vi "TDMS - File Viewer-Custom.vi"(4 "error in (no error)":errorcluster caption="entrée d'erreur (pas d'erreur)", 7 "file path":path caption="chemin du fichier") -> (0 "error out":errorcluster caption="sortie d'erreur", 3 "file path out":path caption="chemin du fichier en sortie")   [LabVIEW 2015]
doc: "<B>Copyright :</B> (c) 2015 National Instruments. Tous droits réservés.\n\nOuvre le fichier .tdms spécifié dans l'entrée <B>chemin du fichier</B> et présente les données du fichier dans la boîte de dialogue TDMS - Afficheur de fichier."
uses:
  <vilib>/Utility/tdmsutil.llb/fileViewerConfigData.ctl
  <vilib>/Utility/error.llb/DialogType.ctl
  <vilib>/event_ctls.llb/sizeaction.ctl
  <vilib>/event_ctls.llb/panelstate.ctl
  <vilib>/Utility/tdmsutil.llb/TDMSFileViewerLocalizedText.vi
  Instance           1 26Saved   TDMS - File Viewer .vi
panel:
  out "LastXScaleFormat":u8 caption="DernierFormatÉchelleX"
  out "TotalCount":u64 caption="Total"
  out "Temp Configuration":T1 caption="Configuration temp."
  in  "LastTopLeftValue":u64 caption="DernièreValeurSupGauche"
  out "Resize?":bool caption="Redimensionner ?"
  in  "Help":bool caption="Aide"
  in  "Status":string caption="État"
  in  "Quit":bool caption="Quitter"
  in  "Settings...":bool caption="Paramètres..."
  in  "Properties / Values / Graph":T2(tab) caption="Propriétés / Valeurs / Graphe"
  in  "Properties":i32(listbox) caption="Propriétés"
  in  "Go To":bool caption="Atteindre"
  in  "Scrollbar":u64(c297) caption="Barre de défilement"
  in  "Raw data values":i32(listbox) caption="Valeurs des données brutes"
  out "Waveform Graph":waveform(dbl)[](graph) caption="Graphe"
  in  "File contents":string(tree) caption="Contenu du fichier"
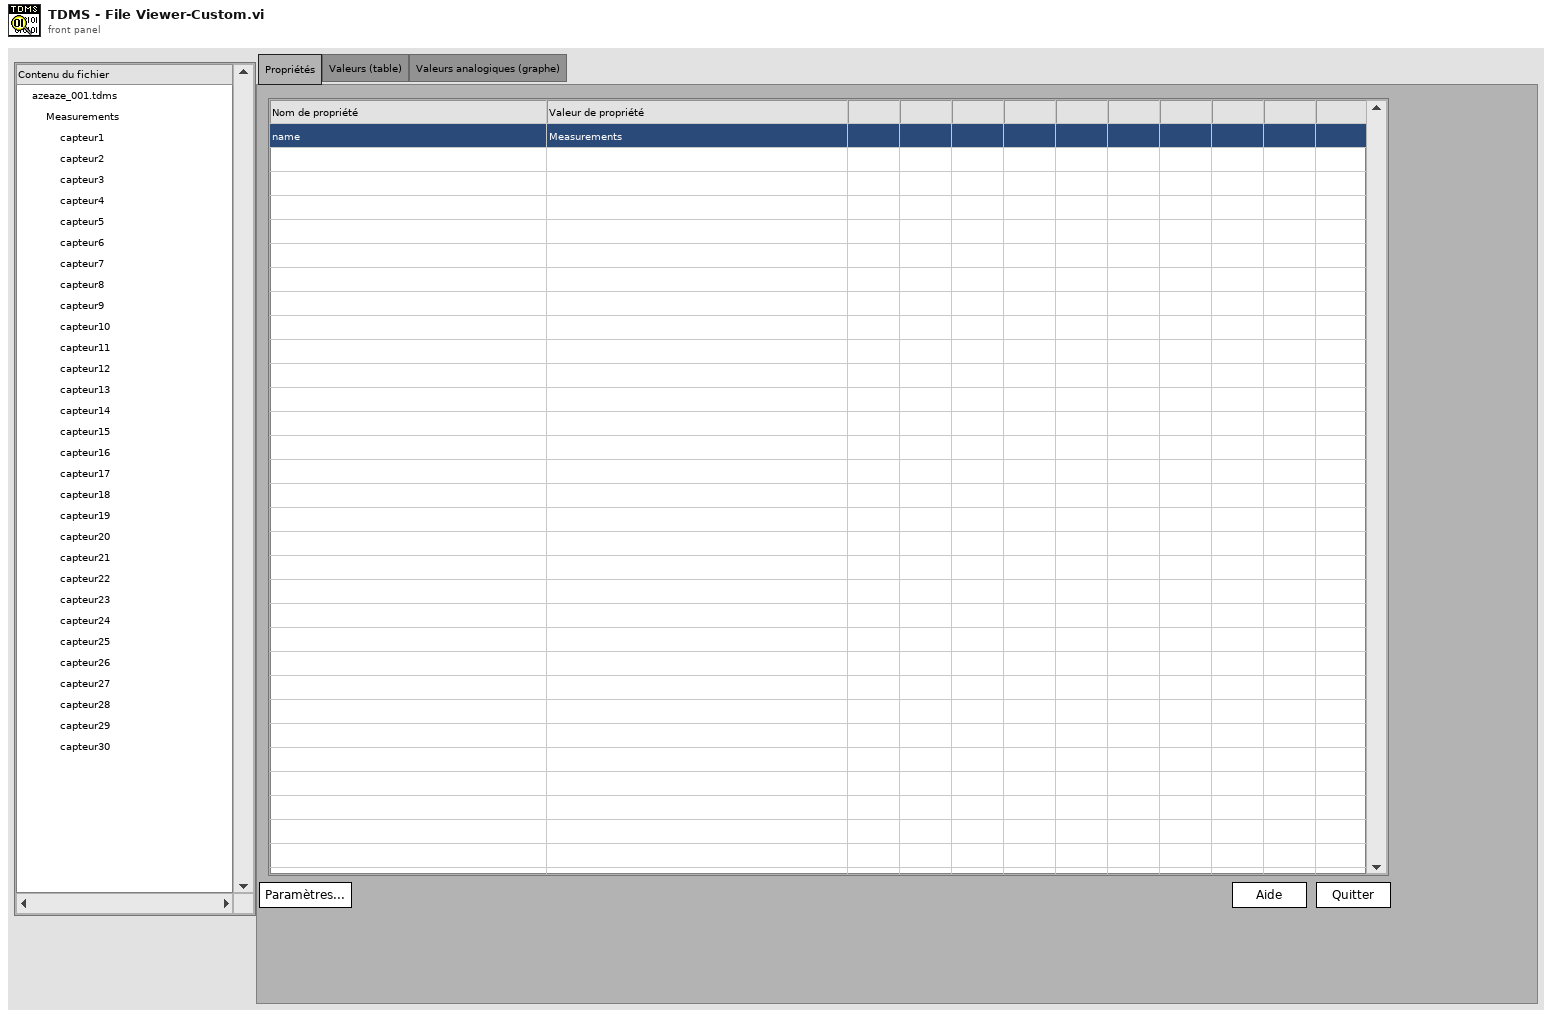
[diagram p1: front panel]
types:
  T1 = typedef "fileViewerConfigData.ctl" = cluster{"Show all (table)":bool, "Show all (graph)":bool, "limit (table)":u64, "limit (graph)":u64, "no show":bool, "start (table)":u64, "start (graph)":u64}
  T2 = enum32{"Properties", "Values (table)", "Analog values (graph)"}
  T3 = enum16{"open", "open or create", "create or replace", "create", "open (read-only)"}
  T4 = cluster{"Tree":refnum<vi>, "Tab Control":refnum<vi>, "property list":refnum<vi>, "raw data list":refnum<vi>, "Waveform Graph":refnum<vi>, "Ok":refnum<vi>, "Ok 2":refnum<vi>, "Ok 3":refnum<vi>, "Ok 4":refnum<vi>, "Scrollbar":refnum<vi>, "Ok 5":refnum<vi>, "TopLeftValue":refnum<vi>, "TotalCount":refnum<vi>}
  T5 = typedef "panelstate.ctl" = enum32{"Standard", "Minimized", "Maximized"}
  T6 = typedef "sizeaction.ctl" = enum32{"Minimized", "Maximized", "Resized"}
  T7 = cluster{"Shift":bool, "Ctrl":bool, "Alt":bool, "Cmd":bool, "Opt":bool}
  T8 = typedef "LVRectTypeDef.ctl" = cluster{"Left":i16, "Top":i16, "Right":i16, "Bottom":i16}
  T9 = typedef "LVRowAndColumnUnsignedTypeDef.ctl" = cluster{"Row":u32, "Column":u32}
  T10 = typedef "DialogType.ctl" = u16
  T11 = typedef "eventvkey.ctl" = enum16{"ASCII", "Enter", "Return", "Shift", "Ctrl", "Alt", "Cmd", "Opt", "Caps", "NumLock", "Clear", "Break", "Up", "Down", "Left", "Right", "Insert", "Delete", "Home", "End", "PageUp", "PageDown", "Escape", "Help", "Pause", "ScrollLock", "F1", "F2", "F3", "F4", "F5", "F6", "F7", "F8", "F9", "F10", "F11", "F12", "F13", "F14", "F15", "F16", "F17", "F18", "F19", "F20", "F21", "F22", "F23", "F24", "Play", "VolumeUp", "VolumeDown", "Mute", "Two Byte Char"}
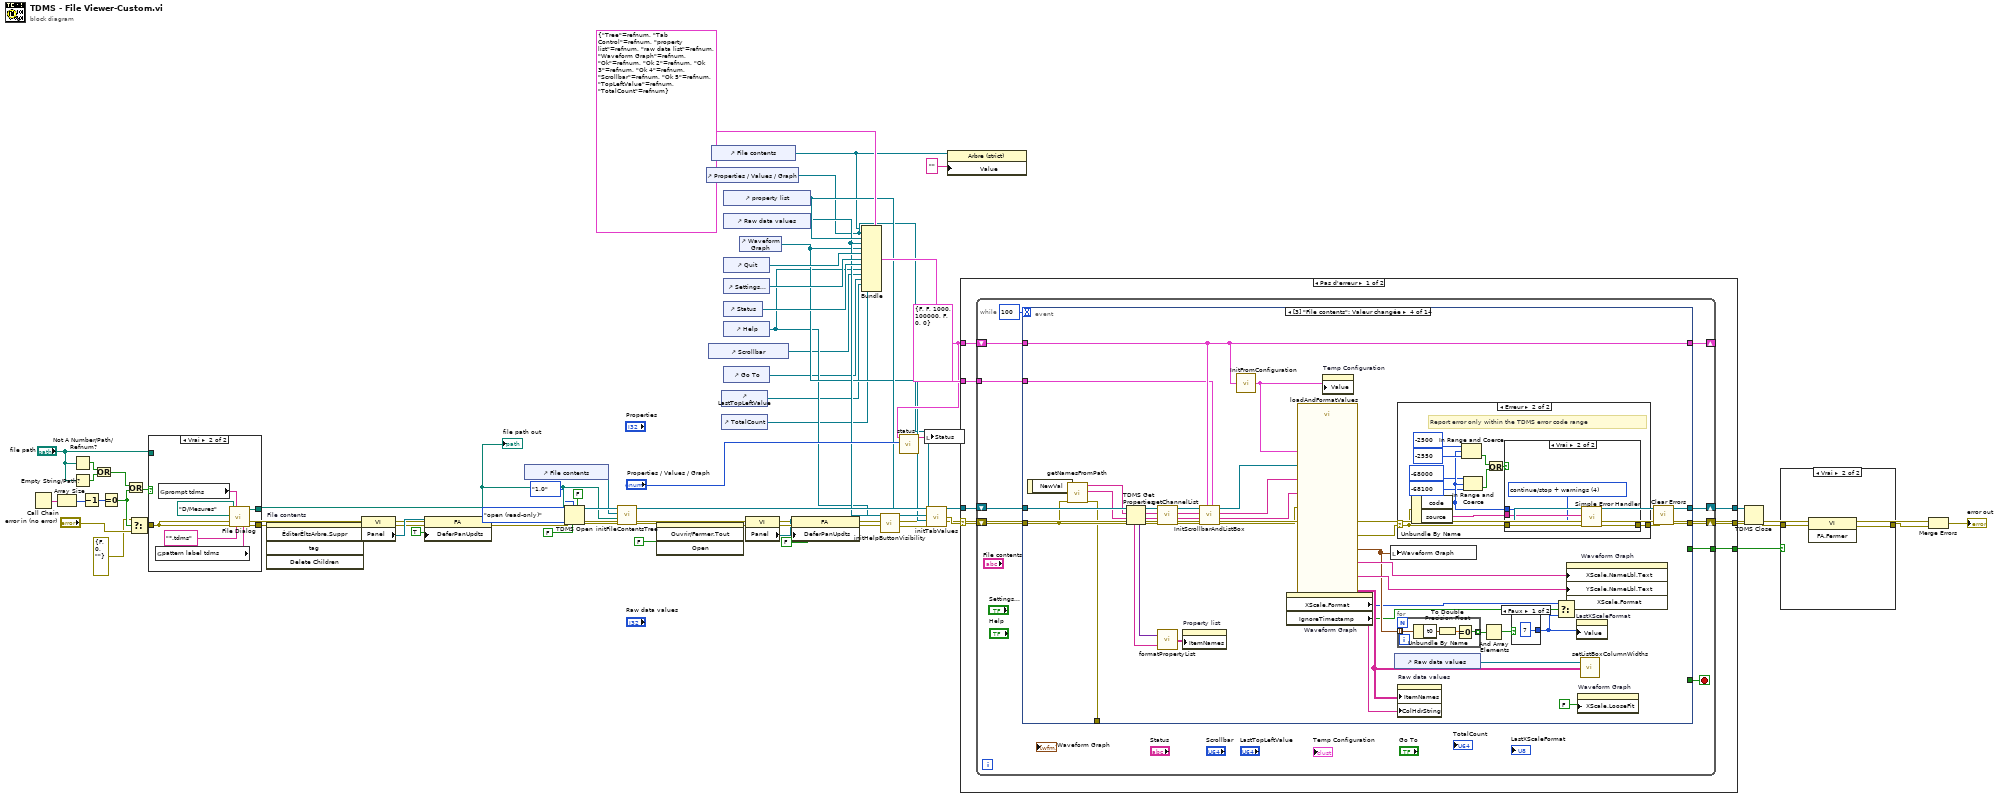
[diagram p0: block diagram]
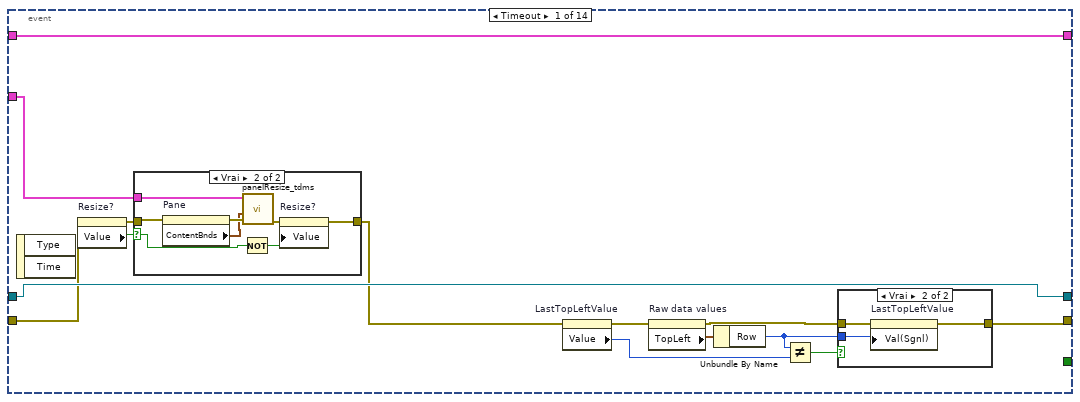
[diagram p3: hidden frame]
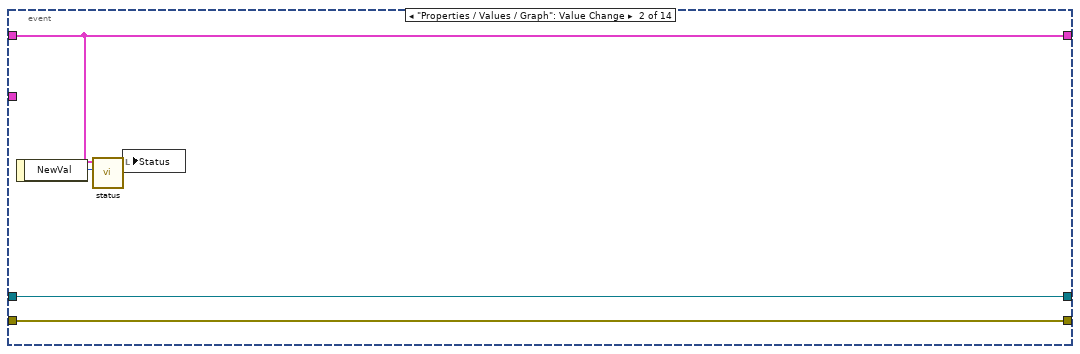
[diagram p6: hidden frame]
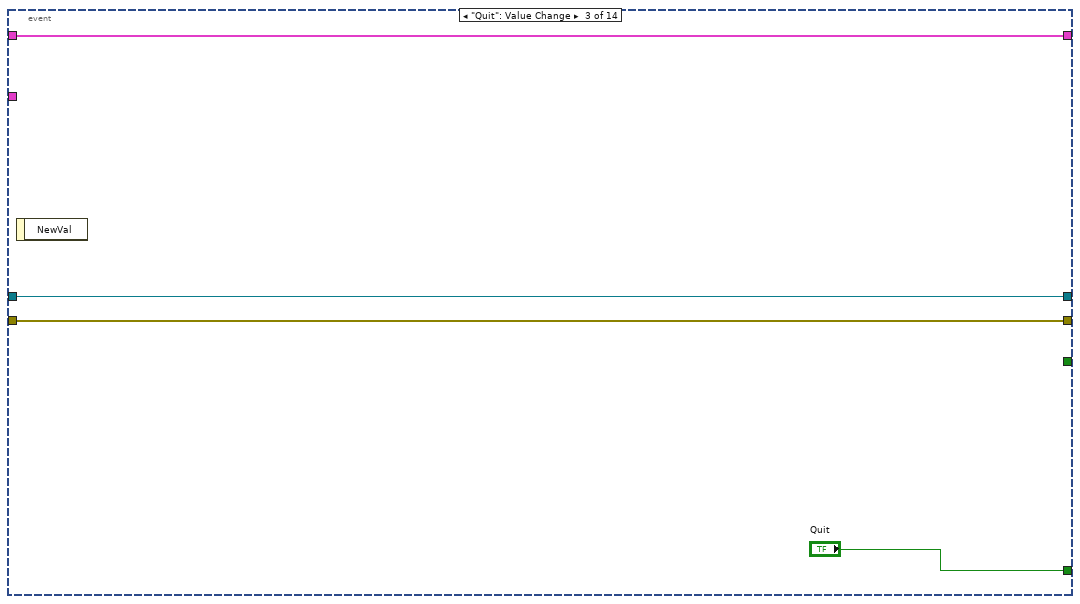
[diagram p7: hidden frame]
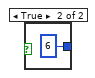
[diagram p8: hidden frame]
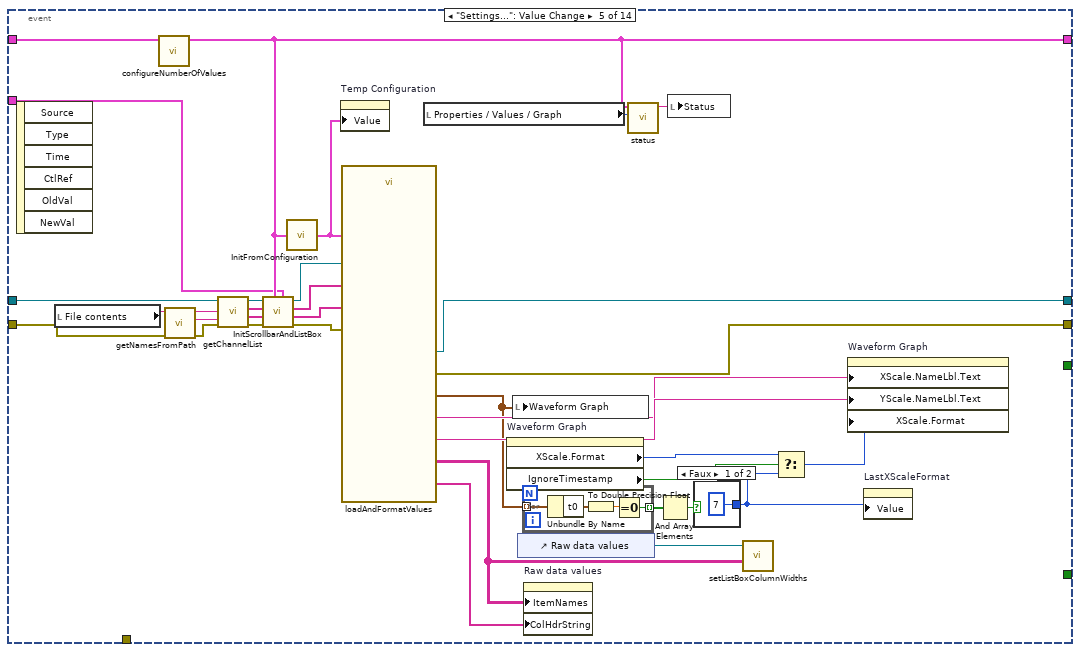
[diagram p11: hidden frame]
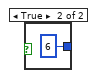
[diagram p12: hidden frame]
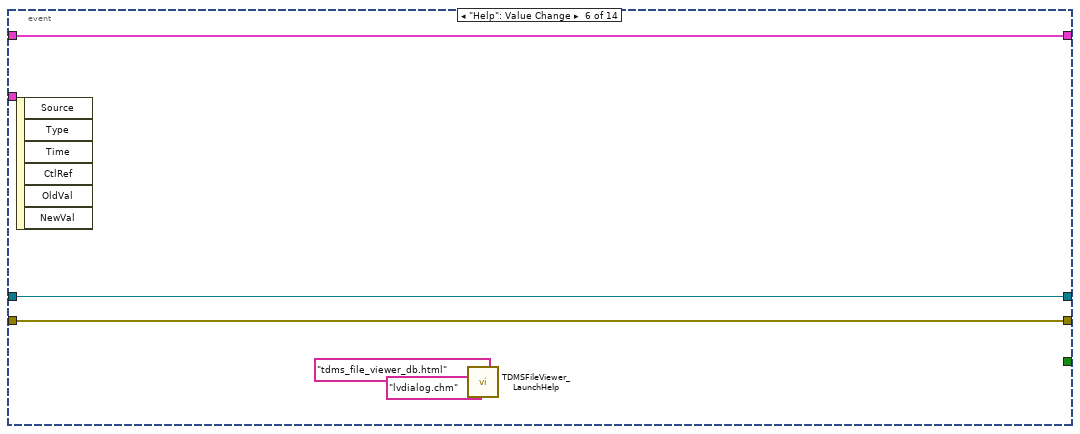
[diagram p13: hidden frame]
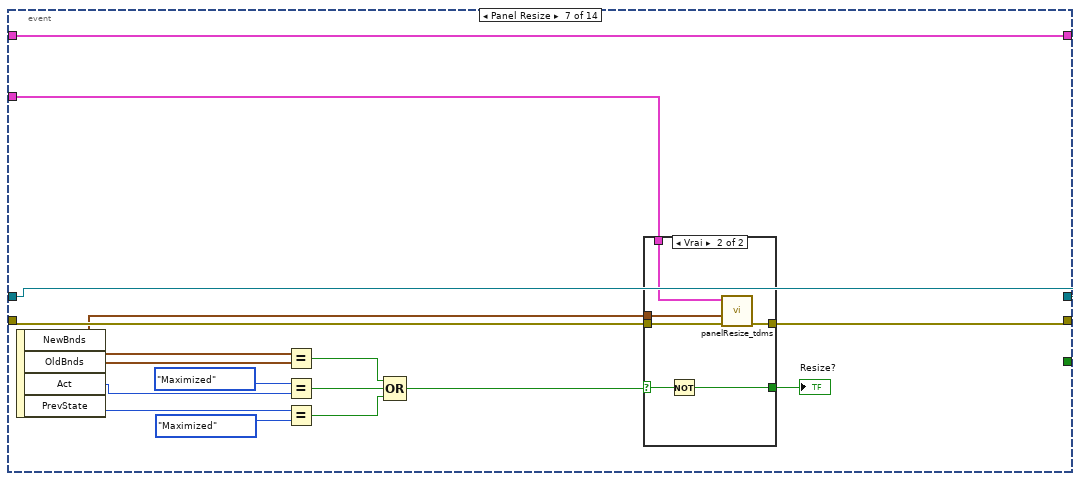
[diagram p14: hidden frame]
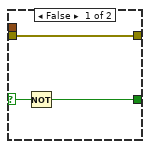
[diagram p15: hidden frame]
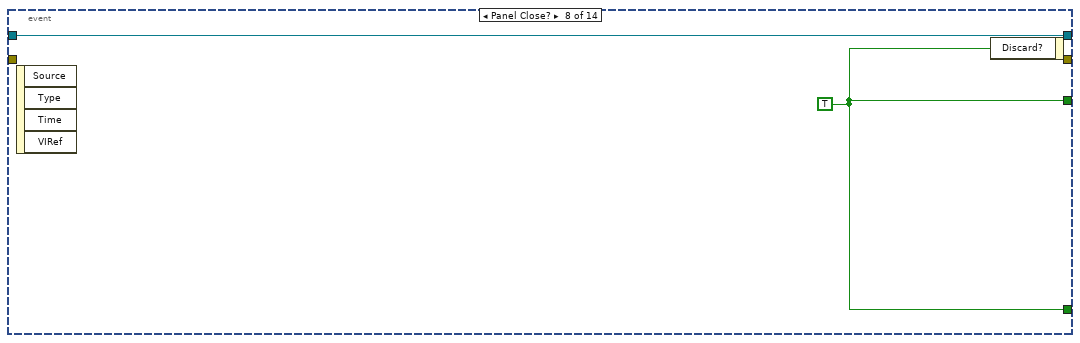
[diagram p16: hidden frame]
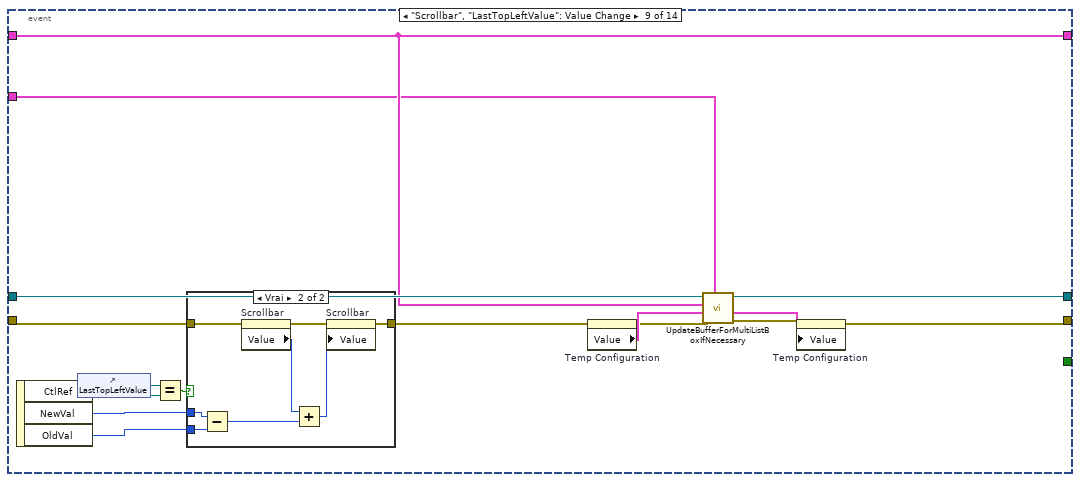
[diagram p17: hidden frame]
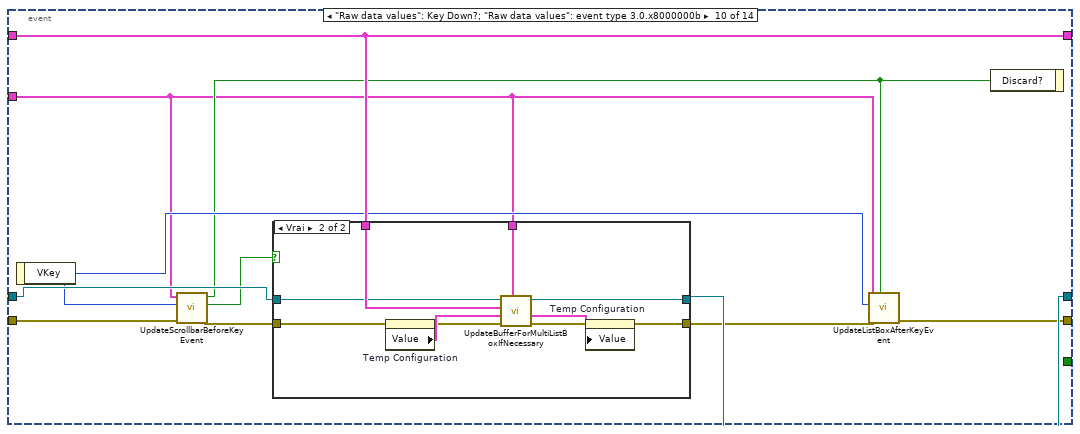
[diagram p19: hidden frame]
diagram:
  w27 = T1 {"Show all (table)"=FALSE, "Show all (graph)"=FALSE, "limit (table)"=1000, "limit (graph)"=100000, "no show"=FALSE, "start (table)"=0, "start (graph)"=0} ("TDMS File Viewer Configuration")
  n1 = Call Chain() -> (call chain=w42:string[])
  n2 = Array Size(array=w42) -> (size(s)=w40:i32)
  n3 = Not A Number/Path/Refnum?(number/path/refnum="file path") -> (NaN/Path/Refnum?=w44:bool)
  n4 = Empty String/Path?(string/path="file path") -> (empty?=w43:bool)
  n5 = Decrement(x=w40) -> (x-1=w39:i32)
  n6 = Or(x=w44, y=w43) -> (x .or. y?=w41:bool)
  n7 = Equal To 0?(x=w39) -> (x = 0?=w25:bool)
  n8 = Or(x=w41, y=w25) -> (x .or. y?=w38:bool)
  n9 = Select(t=errorcluster {"status"=FALSE, "code"=0, "source"=""}, s=w25, f="error in (no error)") -> (s? t:f=w6:errorcluster)
  n10 = case shown="Vrai" w38 {
    tunnel: [w63 w70] -> w31
    tunnel: "file path" -> [w63 _]
    tunnel: [w62 w68] -> w30
    tunnel: w6 -> [w62 w67]
    frame False {
    }
    frame True {
      n11 = global read "TDMSFileViewerLocalizedText.vi" "pattern label tdms"() -> (w65:string)
      n12 = global read "TDMSFileViewerLocalizedText.vi" "prompt tdms"() -> (w66:string)
      n13 = call "File Dialog"("start path"=path "D:/Mesures", "prompt"=w66, "error in"=w67, "pattern (all files)"="*.tdms", "pattern label"=w65) -> ("selected path"=w70:path, "error out"=w68:errorcluster)  [unwired: 2 in, 7 out]
    }
  }
  "file path out" <- w31
  n14 = invoke on="File contents" class="Tree (strict)" method="ÉditerÉltsArbre.Suppr"(error in=w30) -> (error out=w52:errorcluster)  [unwired: 4 in, 4 out]
  n15 = property class="VI"(error in=w52) -> (error out=w53:errorcluster, "Panel"=w54:refnum<vi>)  [unwired: 1 in, 1 out]
  n16 = property class="FA"(reference=w54, error in=w53, "DeferPanUpdts"=TRUE ("Defer Panel Updates")) -> (error out=w56:errorcluster)  [unwired: 1 out]
  n17 = control-ref of="File contents"() -> (w32:refnum<vi>)
  n18 = TDMS Open(5:FALSE ("create index file? (T)"), 6:FALSE ("disable buffering (T)"), 7:enum16{"1.0", "2.0"}."1.0" ("file format version (2.0)"), 8:w56, 10:T3."open (read-only)" ("operation"), 11:w31) -> (0:w61:errorcluster, 3:w60:refnum<k34>)  [unwired: 1 in]
  n19 = call <vilib>:"initFileContentsTree.vi"("error in (no error)"=w61, "file path"=w31, "Tree Refnum"=w32, "tdms file"=w60) -> ("error out"=w48:errorcluster, "tdms file out"=w59:refnum<k34>)  [unwired: 2 out]
  n20 = invoke on="File contents" class="Tree (strict)" method="Ouvrir/Fermer.Tout"(error in=w48, "Open"=FALSE ("Open?")) -> (error out=w47:errorcluster)  [unwired: 2 in, 3 out]
  n21 = control-ref of="Properties / Values / Graph"() -> (w14:refnum<vi>)
  n22 = control-ref of="Scrollbar"() -> (w5:refnum<vi>)
  n23 = control-ref of="File contents"() -> (w13:refnum<vi>)
  n24 = control-ref of="LastTopLeftValue"() -> (w3:refnum<vi>)
  n25 = control-ref of="TotalCount"() -> (w2:refnum<vi>)
  n26 = control-ref of="Status"() -> (w29:refnum<vi>)
  n27 = control-ref of="property list"() -> (w17:refnum<vi>)
  n28 = control-ref of="Raw data values"() -> (w16:refnum<vi>)
  n29 = control-ref of="Quit"() -> (w36:refnum<vi>)
  n30 = control-ref of="Settings..."() -> (w34:refnum<vi>)
  n31 = control-ref of="Help"() -> (w9:refnum<vi>)
  n32 = control-ref of="Go To"() -> (w4:refnum<vi>)
  n33 = control-ref of="Waveform Graph"() -> (w15:refnum<vi>)
  n34 = property class="VI"(error in=w47) -> (error out=w50:errorcluster, "Panel"=w49:refnum<vi>)  [unwired: 1 in, 1 out]
  n35 = property class="FA"(reference=w49, error in=w50, "DeferPanUpdts"=FALSE ("Defer Panel Updates")) -> (error out=w11:errorcluster)  [unwired: 1 out]
  n36 = Bundle(cluster=T4 {"Tree"=refnum, "Tab Control"=refnum, "property list"=refnum, "raw data list"=refnum, "Waveform Graph"=refnum, "Ok"=refnum, "Ok 2"=refnum, "Ok 3"=refnum, "Ok 4"=refnum, "Scrollbar"=refnum, "Ok 5"=refnum, "TopLeftValue"=refnum, "TotalCount"=refnum} ("control refs"), "Tree"=w13, "Tab Control"=w14, "property list"=w17, "raw data list"=w16, "Waveform Graph"=w15, "Ok"=w36, "Ok 2"=w34, "Ok 3"=w29, "Ok 4"=w9, "Scrollbar"=w5, "Ok 5"=w4, "TopLeftValue"=w3, "TotalCount"=w2) -> (w37:T4)
  n37 = call <vilib>:"initHelpButtonVisibility.vi"("error in"=w11, "Help"=w9) -> ("error out"=w10:errorcluster)  [unwired: 9 in]
  n38 = call <vilib>:"status.vi"("tab sheet"="Properties / Values / Graph", "TDMS File Viewer Configuration"=w27) -> ("status"=w28:string)  [unwired: 5 out]
  n39 = local write "Status"(w28) -> ()
  n40 = call <vilib>:"initTabValues.vi"("properties"=w17, "Values"=w16, "waveform"=w15, "error in"=w10, "Properties / Values / Graph"=w14) -> ("error out"=w18:errorcluster)
  n41 = property class="Arbre (strict)"(reference=w13, "Value"="") -> ()  [unwired: 1 in, 2 out]
  n42 = case shown="Pas d'erreur" w18 {
    selector: w18 -> [w72 w394]
    tunnel: w59 -> [w77 w395]
    tunnel: [w76 w395] -> w58
    tunnel: [w75 w393] -> w57
    tunnel: w37 -> [w74 _]
    tunnel: w27 -> [w73 _]
    tunnel: [w71 FALSE] -> w22
    frame No Error {
      n43 = while {
        shift-right: [w85] -> w75
        shift-left: w72 -> [w86]
        shift-right: [w84] -> w76
        shift-left: w77 -> [w87]
        tunnel: w74 -> [w82]
        shift-right: [w80] -> _
        shift-left: w73 -> [w81]
        tunnel: [w79] -> w71
        stop <- w83 stop-if-true
        n44 = event shown="[3] \"File contents\": Valeur changée" {
          selector: _ -> [_ _ _ _ _ _ _ _ _ _ _ _ _ _]
          dyn-events: _ -> [_ _ _ _ _ _ _ _ _ _ _ _ _ _]
          timeout: 100 -> [_ _ _ _ _ _ _ _ _ _ _ _ _ _]
          tunnel: w87 -> [w101 w118 w122 w164 w212 w232 w249 w260 w276 w295 w320 w335 w368 w385]
          tunnel: w86 -> [w96 w119 w121 w156 w219 w231 w247 _ w263 w287 w309 w332 w367 w384]
          tunnel: [w89 w119 w121 w152 w220 w231 w246 _ w270 w292 w312 w333 w367 w376] -> w85
          tunnel: [w101 w118 w122 w163 w221 w232 w249 w260 w275 w294 w319 w334 w368 w385] -> w84
          tunnel: [_ _ "Quit" _ _ _ _ w259 _ _ _ _ _ _] -> w83
          tunnel: [_ _ _ w155 _ _ _ _ _ _ _ _ _ _] -> _
          tunnel: w82 -> [w97 _ _ w131 w196 _ w248 _ w262 w288 w310 w329 _ _]
          tunnel: w81 -> [w100 w115 w120 w132 w222 w233 w245 _ w274 w296 w321 w336 w369 w386]
          tunnel: [w100 w115 w120 w132 w198 w233 w245 _ w274 w296 w321 w336 w369 w386] -> w80
          tunnel: [_ _ _ _ _ _ _ w259 _ _ _ _ _ _] -> w79
          event Timeout {
            n45 = event-data() -> ()  [unwired: 3 out]
            n46 = property on="Resize?" class="Bool (strict)"(error in=w96) -> (error out=w98:errorcluster, "Value"=w99:bool)  [unwired: 1 in, 1 out]
            n47 = case shown="Vrai" w99 {
              selector: w99 -> [_ w113]
              tunnel: w97 -> [_ w114]
              tunnel: w98 -> [w106 w109]
              tunnel: [w106 w111] -> w94
              frame False {
              }
              frame True {
                n48 = property on="Pane" class="Pann"(error in=w109) -> (error out=w108:errorcluster, "ContentBnds"=w107:T8)  [unwired: 1 in, 1 out]
                n49 = Not(x=w113) -> (.not. x?=w110:bool)
                n50 = call <vilib>:"panelResize_tdms.vi"("error in (no error)"=w108, "NewBnds"=w107, "control refs"=w114) -> ("error out"=w112:errorcluster)  [unwired: 4 in]
                n51 = property on="Resize?" class="Bool (strict)"(error in=w112, "Value"=w110) -> (error out=w111:errorcluster)  [unwired: 1 in, 1 out]
              }
            }
            n52 = property on="LastTopLeftValue" class="NumNb (strict)"(error in=w94) -> (error out=w93:errorcluster, "Value"=w92:u64)  [unwired: 1 in, 1 out]
            n53 = property on="Raw data values" class="ListeMCol (strict)"(error in=w93) -> (error out=w90:errorcluster, "TopLeft"=w95:T9)  [unwired: 1 in, 1 out]
            n54 = Unbundle By Name(w95) -> ("Row"=w88:u32)
            n55 = Not Equal?(x=w88, y=w92) -> (x != y?=w91:bool)
            n56 = case shown="Vrai" w91 {
              tunnel: w90 -> [w102 w105]
              tunnel: [w102 w104] -> w89
              tunnel: w88 -> [_ w103]
              frame False {
              }
              frame True {
                n57 = property on="LastTopLeftValue" class="NumNb (strict)"(error in=w105, "Val(Sgnl)"=w103) -> (error out=w104:errorcluster)  [unwired: 1 in, 1 out]
              }
            }
          }
          event "Properties / Values / Graph": Value Change {
            n58 = event-data() -> ("NewVal"=w117:T2)  [unwired: 1 out]
            n59 = call <vilib>:"status.vi"("tab sheet"=w117, "TDMS File Viewer Configuration"=w115) -> ("status"=w116:string)  [unwired: 5 out]
            n60 = local write "Status"(w116) -> ()
          }
          event "Quit": Value Change {
            n61 = event-data() -> ()  [unwired: 2 out]
          }
          event "File contents": Value Change {
            n62 = event-data() -> ("NewVal"=w158:string)  [unwired: 1 out]
            n63 = call <vilib>:"getNamesFromPath.vi"("error in (no error)"=w156, "tree path"=w158) -> ("error out"=w155:errorcluster, "channel"=w161:string, "group"=w162:string)  [unwired: 3 out]
            n64 = TDMS Get Properties(8:w156, 9:w161, 10:w162, 11:w164) -> (0:w150:errorcluster, 1:w149:string, 2:w145:string, 3:w151:refnum<k34>, 4:w159:variant[], 6:w160:string[])  [unwired: 2 out]
            n65 = call <vilib>:"getChannelList.vi"("error in (no error)"=w150, "channel names"=w149, "group name"=w145, "tdms file"=w151) -> ("error out"=w140:errorcluster, "channel names out"=w138:string[], "group names out"=w136:string[], "tdms file out"=w134:refnum<k34>)
            n66 = call <vilib>:"formatPropertyList.vi"("property names"=w160, "property values"=w159) -> ("strings"=w157:string[][])
            n67 = property on="Property list" class="ListeMCol (strict)"("ItemNames"=w157) -> ()  [unwired: 2 in, 2 out]
            n68 = call <vilib>:"InitScrollbarAndListBox.vi"("control refs"=w131, "configuration"=w132, "error in (no error)"=w140, "channel names"=w138, "group names"=w136, "tdms in"=w134) -> ("error out"=w139:errorcluster, "channel out"=w137:string[], "group out"=w135:string[], "tdms out"=w133:refnum<k34>)  [unwired: 2 in]
            n69 = call <vilib>:"InitFromConfiguration.vi"("configuration"=w132) -> ("output cluster"=w141:T1)  [unwired: 4 in]
            n70 = property on="Waveform Graph" class="GraphWF (strict)"() -> ("XScale.Format"=w125:u8, "IgnoreTimestamp"=w124:bool)  [unwired: 2 in, 2 out]
            n71 = call <vilib>:"loadAndFormatValues.vi"("error in (no error)"=w139, "configuration"=w141, "channel names"=w137, "group names"=w135, "tdms file"=w133) -> ("error out"=w144:errorcluster, "graph y names"=w147:string, "graph x names"=w146:string, "tdms file out"=w163:refnum<k34>, "waveform values"=w130:waveform(dbl)[], "table values"=w154:string[][], "table headers"=w148:string[])
            n72 = property on="Temp Configuration" class="Clust (strict)"("Value"=w141) -> ()  [unwired: 2 in, 2 out]
            n73 = local write "Waveform Graph"(w130) -> ()
            n74 = control-ref of="Raw data values"() -> (w153:refnum<vi>)
            n75 = case shown="Erreur" w144 {
              selector: w144 -> [w171 w181]
              tunnel: [w171 w180] -> w143
              frame No Error {
              }
              frame Error {
                # "Report error only within the TDMS error code range"
                n76 = Unbundle By Name(w181) -> ("code"=w177:i32, "source"=w182:string)
                n77 = In Range and Coerce(upper limit=-2500, x=w177, lower limit=-2550 ("upper limit")) -> (In Range?=w174:bool)  [unwired: 1 out]
                n78 = In Range and Coerce(upper limit=-68000, x=w177, lower limit=-68100) -> (In Range?=w173:bool)  [unwired: 1 out]
                n79 = Or(x=w174, y=w173) -> (x .or. y?=w172:bool)
                n80 = case shown="Vrai" w172 {
                  tunnel: w182 -> [_ w188]
                  tunnel: w181 -> [w183 w187]
                  tunnel: [w183 w186] -> w180
                  tunnel: w177 -> [_ w184]
                  frame False {
                    # "Out of the range of TDMS\nerror code, we don't report\nthem."
                  }
                  frame True {
                    w185 = T10 4 items=["no dialog", "OK message", "continue or stop message", "OK message + warnings", "continue/stop + warnings"] ("type of dialog (OK msg:1)")
                    n81 = call <vilib>:"Simple Error Handler.vi"("error code (no error:0)"=w184, "error source (\" \")"=w188, "type of dialog (OK msg:1)"=w185, "error in (no error)"=w187) -> ("error out"=w186:errorcluster)  [unwired: 1 in, 4 out]
                  }
                }
              }
            }
            n82 = for {
              tunnel: w130 -> [w170] mode=indexing
              tunnel: [w167] -> w129 mode=indexing
              n83 = Unbundle By Name(w170) -> ("t0"=w169:timestamp)
              n84 = To Double Precision Float(number=w169) -> (double precision float=w168:dbl)
              n85 = Equal To 0?(x=w168) -> (x = 0?=w167:bool)
            }
            n86 = property on="Raw data values" class="ListeMCol (strict)"("ItemNames"=w154, "ColHdrString"=w148) -> ()  [unwired: 2 in, 2 out]
            n87 = And Array Elements(Boolean array=w129) -> (logical AND=w128:bool)
            n88 = case shown="Faux" w128 {
              tunnel: [u8 7 u8 6] -> w126
              frame False {
              }
              frame True {
              }
            }
            n89 = Select(t=w125, s=w124, f=w126) -> (s? t:f=w127:u8)
            n90 = property on="Waveform Graph" class="GraphWF (strict)"("XScale.NameLbl.Text"=w146, "YScale.NameLbl.Text"=w147, "XScale.Format"=w127) -> ()  [unwired: 2 in, 2 out]
            n91 = property on="LastXScaleFormat" class="NumNb (strict)"("Value"=w126) -> ()  [unwired: 2 in, 2 out]
            n92 = property on="Waveform Graph" class="GraphWF (strict)"("XScale.LooseFit"=FALSE ("X Scale.Loose Fit")) -> ()  [unwired: 2 in, 2 out]
            n93 = call <vilib>:"setListBoxColumnWidths.vi"("table data"=w154, "MCListbox Refnum"=w153) -> ()  [unwired: 1 out]
            n94 = call <vilib>:"Clear Errors.vi"("error in (no error)"=w143) -> ("error out"=w152:errorcluster)  [unwired: 1 in, 5 out]
          }
          event "Settings...": Value Change {
            n95 = event-data() -> ()  [unwired: 7 out]
            n96 = local read "File contents"() -> (w213:string)
            n97 = call <vilib>:"configureNumberOfValues.vi"("TDMS File Viewer Configuration"=w222) -> ("TDMS File Viewer Configuration Out"=w198:T1)  [unwired: 10 out]
            n98 = call <vilib>:"getNamesFromPath.vi"("error in (no error)"=w219, "tree path"=w213) -> ("error out"=w211:errorcluster, "channel"=w209:string, "group"=w210:string)  [unwired: 3 out]
            n99 = call <vilib>:"getChannelList.vi"("error in (no error)"=w211, "channel names"=w209, "group name"=w210, "tdms file"=w212) -> ("error out"=w200:errorcluster, "channel names out"=w202:string[], "group names out"=w204:string[], "tdms file out"=w206:refnum<k34>)
            n100 = call <vilib>:"InitScrollbarAndListBox.vi"("control refs"=w196, "configuration"=w198, "error in (no error)"=w200, "channel names"=w202, "group names"=w204, "tdms in"=w206) -> ("error out"=w199:errorcluster, "channel out"=w201:string[], "group out"=w203:string[], "tdms out"=w205:refnum<k34>)  [unwired: 2 in]
            n101 = call <vilib>:"InitFromConfiguration.vi"("configuration"=w198) -> ("output cluster"=w197:T1)  [unwired: 4 in]
            n102 = property on="Temp Configuration" class="Clust (strict)"("Value"=w197) -> ()  [unwired: 2 in, 2 out]
            n103 = call <vilib>:"loadAndFormatValues.vi"("error in (no error)"=w199, "configuration"=w197, "channel names"=w201, "group names"=w203, "tdms file"=w205) -> ("error out"=w220:errorcluster, "graph y names"=w215:string, "graph x names"=w214:string, "tdms file out"=w221:refnum<k34>, "waveform values"=w193:waveform(dbl)[], "table values"=w216:string[][], "table headers"=w218:string[])
            n104 = local read "Properties / Values / Graph"() -> (w207:T2)
            n105 = property on="Waveform Graph" class="GraphWF (strict)"() -> ("XScale.Format"=w190:u8, "IgnoreTimestamp"=w189:bool)  [unwired: 2 in, 2 out]
            n106 = local write "Waveform Graph"(w193) -> ()
            n107 = control-ref of="Raw data values"() -> (w217:refnum<vi>)
            n108 = for {
              tunnel: w193 -> [w228] mode=indexing
              tunnel: [w225] -> w195 mode=indexing
              n109 = Unbundle By Name(w228) -> ("t0"=w227:timestamp)
              n110 = To Double Precision Float(number=w227) -> (double precision float=w226:dbl)
              n111 = Equal To 0?(x=w226) -> (x = 0?=w225:bool)
            }
            n112 = property on="Raw data values" class="ListeMCol (strict)"("ItemNames"=w216, "ColHdrString"=w218) -> ()  [unwired: 2 in, 2 out]
            n113 = call <vilib>:"status.vi"("tab sheet"=w207, "TDMS File Viewer Configuration"=w198) -> ("status"=w208:string)  [unwired: 5 out]
            n114 = And Array Elements(Boolean array=w195) -> (logical AND=w194:bool)
            n115 = local write "Status"(w208) -> ()
            n116 = case shown="Faux" w194 {
              tunnel: [u8 7 u8 6] -> w191
              frame False {
              }
              frame True {
              }
            }
            n117 = call <vilib>:"setListBoxColumnWidths.vi"("table data"=w216, "MCListbox Refnum"=w217) -> ()  [unwired: 1 out]
            n118 = Select(t=w190, s=w189, f=w191) -> (s? t:f=w192:u8)
            n119 = property on="Waveform Graph" class="GraphWF (strict)"("XScale.NameLbl.Text"=w214, "YScale.NameLbl.Text"=w215, "XScale.Format"=w192) -> ()  [unwired: 2 in, 2 out]
            n120 = property on="LastXScaleFormat" class="NumNb (strict)"("Value"=w191) -> ()  [unwired: 2 in, 2 out]
          }
          event "Help": Value Change {
            n121 = event-data() -> ()  [unwired: 7 out]
            n122 = call <vilib>:"TDMSFileViewer_LaunchHelp.vi"("CHM or HLP filename (lvdialog.chm)"="lvdialog.chm", "HTML filename"="tdms_file_viewer_db.html") -> ()  [unwired: 1 in, 5 out]
          }
          event Panel Resize {
            n123 = event-data() -> ("NewBnds"=w237:T8, "OldBnds"=w236:T8, "Act"=w238:T6, "PrevState"=w239:T5)  [unwired: 1 out]
            n124 = Equal?(x=w237, y=w236) -> (x = y?=w242:bool)
            n125 = Equal?(x=sizeaction."Maximized" ("Act"), y=w238) -> (x = y?=w241:bool)
            n126 = Equal?(x=w239, y=panelstate."Maximized" ("PrevState")) -> (x = y?=w240:bool)
            n127 = Compound Arithmetic op=OR(w242, w241, w240) -> (w235:bool)
            n128 = case shown="Vrai" w235 {
              selector: w235 -> [w251 w254]
              tunnel: w248 -> [_ w258]
              tunnel: w247 -> [w252 w257]
              tunnel: [w252 w256] -> w246
              tunnel: w237 -> [_ w255]
              tunnel: [w250 w253] -> w234
              frame False {
                n129 = Not(x=w251) -> (.not. x?=w250:bool)
              }
              frame True {
                n130 = Not(x=w254) -> (.not. x?=w253:bool)
                n131 = call <vilib>:"panelResize_tdms.vi"("error in (no error)"=w257, "NewBnds"=w255, "control refs"=w258) -> ("error out"=w256:errorcluster)  [unwired: 4 in]
              }
            }
            "Resize?" <- w234
          }
          event Panel Close? {
            w259 = TRUE
            n132 = event-data() -> ()  [unwired: 5 out]
            n133 = event-data("Discard?"=w259) -> ()  [unwired: 1 in, 1 out]
          }
          event "Scrollbar", "LastTopLeftValue": Value Change {
            n134 = event-data() -> ("CtlRef"=w268:refnum<vi>, "NewVal"=w265:u64, "OldVal"=w264:u64)  [unwired: 1 out]
            n135 = control-ref of="LastTopLeftValue"() -> (w267:refnum<vi>)
            n136 = Equal?(x=w267, y=w268) -> (x = y?=w266:bool)
            n137 = case shown="Vrai" w266 {
              tunnel: w265 -> [_ w281]
              tunnel: w264 -> [_ w280]
              tunnel: w263 -> [w277 w279]
              tunnel: [w277 w278] -> w261
              frame False {
              }
              frame True {
                n138 = Subtract(x=w281, y=w280) -> (x-y=w283:u64)
                n139 = property on="Scrollbar" class="BarDéf (strict)"(error in=w279) -> (error out=w285:errorcluster, "Value"=w284:u64)  [unwired: 1 in, 1 out]
                n140 = Add(x=w284, y=w283) -> (x+y=w282:u64)
                n141 = property on="Scrollbar" class="BarDéf (strict)"(error in=w285, "Value"=w282) -> (error out=w278:errorcluster)  [unwired: 1 in, 1 out]
              }
            }
            n142 = property on="Temp Configuration" class="Clust (strict)"(error in=w261) -> (error out=w272:errorcluster, "Value"=w273:T1)  [unwired: 1 in, 1 out]
            n143 = call <vilib>:"UpdateBufferForMultiListBoxIfNecessary.vi"("control refs"=w262, "error in"=w272, "Buffer Configuration"=w273, "TDMS File Viewer Configuration"=w274, "tdms file in"=w276) -> ("error out"=w271:errorcluster, "BufferConfig out"=w269:T1, "tdms file out"=w275:refnum<k34>)  [unwired: 4 in]
            n144 = property on="Temp Configuration" class="Clust (strict)"(error in=w271, "Value"=w269) -> (error out=w270:errorcluster)  [unwired: 1 in, 1 out]
          }
          event "Raw data values": Key Down?; "Raw data values": event type 3.0.x8000000b {
            n145 = event-data() -> ("VKey"=w290:T11)  [unwired: 1 out]
            n146 = call <vilib>:"UpdateScrollbarBeforeKeyEvent.vi"("error in (no error)"=w287, "VKey"=w290, "control refs 2"=w288) -> ("error out"=w293:errorcluster, "LoadBuffer?"=w291:bool, "DiscardEvent?"=w289:bool)  [unwired: 6 in]
            n147 = case shown="Vrai" w291 {
              tunnel: w296 -> [_ w304]
              tunnel: w295 -> [w297 w303]
              tunnel: [w297 w302] -> w294
              tunnel: w293 -> [w298 w299]
              tunnel: [w298 w301] -> w286
              tunnel: w288 -> [_ w300]
              frame False {
              }
              frame True {
                n148 = property on="Temp Configuration" class="Clust (strict)"(error in=w299) -> (error out=w307:errorcluster, "Value"=w308:T1)  [unwired: 1 in, 1 out]
                n149 = call <vilib>:"UpdateBufferForMultiListBoxIfNecessary.vi"("control refs"=w300, "error in"=w307, "Buffer Configuration"=w308, "TDMS File Viewer Configuration"=w304, "tdms file in"=w303) -> ("error out"=w306:errorcluster, "BufferConfig out"=w305:T1, "tdms file out"=w302:refnum<k34>)  [unwired: 4 in]
                n150 = property on="Temp Configuration" class="Clust (strict)"(error in=w306, "Value"=w305) -> (error out=w301:errorcluster)  [unwired: 1 in, 1 out]
              }
            }
            n151 = call <vilib>:"UpdateListBoxAfterKeyEvent.vi"("DiscardEvent?"=w289, "error in (no error)"=w286, "VKey"=w290, "control refs"=w288) -> ("error out"=w292:errorcluster)  [unwired: 7 in]
            n152 = event-data("Discard?"=w289) -> ()  [unwired: 1 in, 1 out]
          }
          event "Go To": Value Change {
            n153 = event-data() -> ()  [unwired: 2 out]
            n154 = call <vilib>:"GoTo.vi"("error in"=w309, "control refs"=w310) -> ("error out"=w318:errorcluster, "VisibleValue"=w315:u64)  [unwired: 8 in]
            n155 = property on="Temp Configuration" class="Clust (strict)"(error in=w318) -> (error out=w324:errorcluster, "Value"=w325:T1)  [unwired: 1 in, 1 out]
            n156 = call <vilib>:"UpdateBufferForMultiListBoxIfNecessary.vi"("control refs"=w310, "error in"=w324, "Buffer Configuration"=w325, "TDMS File Viewer Configuration"=w321, "tdms file in"=w320) -> ("error out"=w323:errorcluster, "BufferConfig out"=w322:T1, "tdms file out"=w319:refnum<k34>)  [unwired: 4 in]
            n157 = property on="Temp Configuration" class="Clust (strict)"(error in=w323, "Value"=w322) -> (error out=w311:errorcluster)  [unwired: 1 in, 1 out]
            n158 = property on="Raw data values" class="ListeMCol (strict)"(error in=w311) -> (error out=w313:errorcluster, "TopLeft"=w317:T9)  [unwired: 1 in, 1 out]
            n159 = Unbundle By Name(w317) -> ("Row"=w316:u32)
            n160 = Add(x=w316, y=w315) -> (x+y=w314:u64)
            n161 = property on="Raw data values" class="ListeMCol (strict)"(error in=w313, "Value"=w314) -> (error out=w312:errorcluster)  [unwired: 1 in, 1 out]
          }
          event Key Down {
            n162 = event-data() -> ("PlatMods"=w328:T7, "Char"=w327:i16)  [unwired: 1 out]
            n163 = property on="Raw data values" class="ListeMCol (strict)"(error in=w332) -> (error out=w326:errorcluster, "Key Focus"=w331:bool)  [unwired: 1 in, 1 out]
            n164 = case shown="Vrai" w331 {
              selector: w331 -> [w337 _]
              tunnel: [w337 w338] -> w330
              tunnel: w328 -> [_ w343]
              tunnel: w327 -> [_ w342]
              frame False {
              }
              frame True {
                n165 = disable-structure shown="Default" {
                  disable-tunnel: [T7 {"Shift"=FALSE, "Ctrl"=TRUE, "Alt"=FALSE, "Cmd"=FALSE, "Opt"=TRUE} ("PlatMods") T7 {"Shift"=FALSE, "Ctrl"=FALSE, "Alt"=FALSE, "Cmd"=TRUE, "Opt"=FALSE} ("PlatMods")] -> w344
                  frame condition #0 (active) {
                  }
                  frame condition #1 {
                  }
                }
                n166 = Equal?(x=w344, y=w343) -> (x = y?=w340:bool)
                n167 = Equal?(x=w342, y=i16 103 ("Char")) -> (x = y?=w339:bool)
                n168 = And(x=w340, y=w339) -> (x .and. y?=w338:bool)
              }
            }
            n169 = case shown="Vrai" w330 {
              tunnel: w336 -> [_ w362]
              tunnel: w335 -> [w347 w361]
              tunnel: [w347 w360] -> w334
              tunnel: [w348 w353] -> w333
              tunnel: w326 -> [w348 w349]
              tunnel: w329 -> [_ w351]
              tunnel: w329 -> [_ w350]
              frame False {
              }
              frame True {
                n170 = call <vilib>:"GoTo.vi"("error in"=w349, "control refs"=w350) -> ("error out"=w359:errorcluster, "VisibleValue"=w356:u64)  [unwired: 8 in]
                n171 = property on="Temp Configuration" class="Clust (strict)"(error in=w359) -> (error out=w365:errorcluster, "Value"=w366:T1)  [unwired: 1 in, 1 out]
                n172 = call <vilib>:"UpdateBufferForMultiListBoxIfNecessary.vi"("control refs"=w351, "error in"=w365, "Buffer Configuration"=w366, "TDMS File Viewer Configuration"=w362, "tdms file in"=w361) -> ("error out"=w364:errorcluster, "BufferConfig out"=w363:T1, "tdms file out"=w360:refnum<k34>)  [unwired: 4 in]
                n173 = property on="Temp Configuration" class="Clust (strict)"(error in=w364, "Value"=w363) -> (error out=w352:errorcluster)  [unwired: 1 in, 1 out]
                n174 = property on="Raw data values" class="ListeMCol (strict)"(error in=w352) -> (error out=w354:errorcluster, "TopLeft"=w358:T9)  [unwired: 1 in, 1 out]
                n175 = Unbundle By Name(w358) -> ("Row"=w357:u32)
                n176 = Add(x=w357, y=w356) -> (x+y=w355:u64)
                n177 = property on="Raw data values" class="ListeMCol (strict)"(error in=w354, "Value"=w355) -> (error out=w353:errorcluster)  [unwired: 1 in, 1 out]
              }
            }
          }
          event Key Down? {
            n178 = event-data() -> ("VKey"=w371:T11)  [unwired: 1 out]
            n179 = case shown="\"F1\"" w371 {
              tunnel: [FALSE ("Discard?") TRUE ("Discard?")] -> w370
              frame Default {
              }
              frame "F1" {
                n180 = call <vilib>:"TDMSFileViewer_LaunchHelp.vi"("CHM or HLP filename (lvdialog.chm)"="lvdialog.chm", "HTML filename"="tdms_file_viewer_db.html") -> ()  [unwired: 1 in, 5 out]
              }
            }
            n181 = event-data("Discard?"=w370) -> ()  [unwired: 1 in, 1 out]
          }
          event "Waveform Graph": Shortcut Menu Selection (App) {
            n182 = event-data() -> ("ItemTag"=w382:string)  [unwired: 1 out]
            n183 = property on="Waveform Graph" class="GraphWF (strict)"(error in=w384) -> (error out=w377:errorcluster, "IgnoreTimestamp"=w381:bool)  [unwired: 1 in, 1 out]
            n184 = Not(x=w381) -> (.not. x?=w378:bool)
            n185 = Equal?(x=w382, y="APP_SC_IGNORE_TIME_STAMP") -> (x = y?=w379:bool)
            n186 = And(x=w378, y=w379) -> (x .and. y?=w380:bool)
            n187 = case shown="Vrai" w380 {
              tunnel: w377 -> [w387 w391]
              tunnel: [w387 w388] -> w376
              frame False {
              }
              frame True {
                n188 = property on="LastXScaleFormat" class="NumNb (strict)"(error in=w391) -> (error out=w390:errorcluster, "Value"=w389:u8)  [unwired: 1 in, 1 out]
                n189 = property on="Waveform Graph" class="GraphWF (strict)"(error in=w390, "XScale.Format"=w389) -> (error out=w388:errorcluster)  [unwired: 1 in, 1 out]
              }
            }
          }
        }
      }
    }
    frame Error {
      n190 = call <vilib>:"Simple Error Handler.vi"("error in (no error)"=w394) -> ("error out"=w393:errorcluster)  [unwired: 1 in, 7 out]
    }
  }
  n191 = TDMS Close(8:w57, 11:w58) -> (0:w21:errorcluster)  [unwired: 1 out]
  n192 = case shown="Vrai" w22 {
    tunnel: w21 -> [w396 w398]
    tunnel: [w396 w397] -> w8
    frame False {
    }
    frame True {
      n193 = invoke class="VI" method="FA.Fermer"(error in=w398) -> (error out=w397:errorcluster)  [unwired: 2 in, 2 out]
    }
  }
  n194 = Merge Errors(w6, w8) -> (→"error out":errorcluster)
